vi "Or.vi"(1 "b":bool, 2 "a":bool) -> (0 "x":bool)   [LabVIEW 2012]
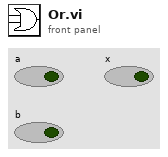
[diagram p1: front panel]
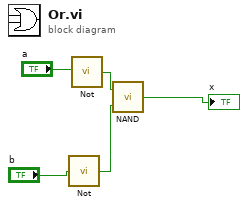
[diagram p0: block diagram]
diagram:
  n1 = call "Not.vi"("In"="b") -> ("Out"=w4:bool)
  n2 = call "Not.vi"("In"="a") -> ("Out"=w3:bool)
  n3 = call "NAND.vi"("b"=w4, "a"=w3) -> ("x"=→"x":bool)
